vi "Field Get Field.vi"(6 "by sDisplayName? (f, by sFieldId)":bool, 7 "Include deleted? (F)":bool, 8 "error in (no error)":errorcluster, 9 "sFieldId or sDisplayName (\"\")":string, 10 "sxSequenceId (\"\")":string, 11 "Connection Refnum":T4) -> (0 "error out":errorcluster, 2 "Field":T1={"ixField"=0, "iSequenceOrder"=0, "sxFieldId"="", "sxSequenceId"="", "sDisplayName"="", "sValue"="", "sUnits"="", "nDataType"=enum."timestamp", "nNextItem"=enum."Reset", "fSystem"=FALSE, "fSystemValue"=FALSE, "fRequired"=FALSE, "fSetAtTest"=FALSE, "fTestField"=FALSE, "fDeleted"=FALSE, "fIndexed"=FALSE, "fFreeList"=FALSE}, 3 "Connection Refnum":T4, 4 "Data Present?":bool)   [LabVIEW 2011]
uses:
  Summitek EXT/ODBC/SQL Controls/Connection Refnum.ctl
  Field Record.ctl
  Field DataTypes.ctl
  Field NextItem.ctl
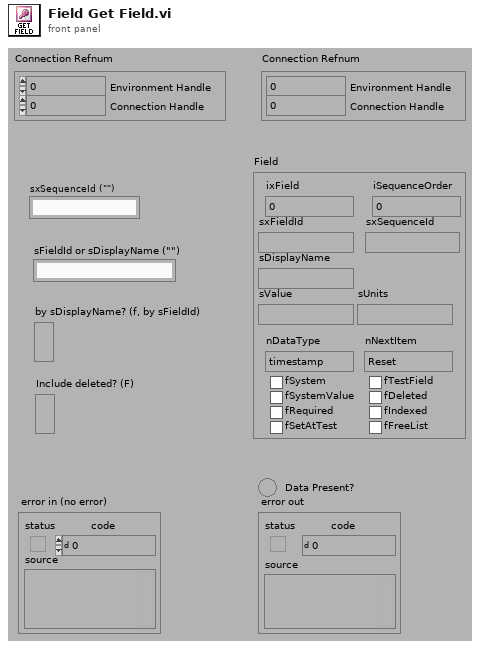
[diagram p1: front panel]
types:
  T1 = typedef "Field Record.ctl" = cluster{"ixField":i32, "iSequenceOrder":i32, "sxFieldId":string, "sxSequenceId":string, "sDisplayName":string, "sValue":string, "sUnits":string, "nDataType":T2, "nNextItem":T3, "fSystem":bool, "fSystemValue":bool, "fRequired":bool, "fSetAtTest":bool, "fTestField":bool, "fDeleted":bool, "fIndexed":bool, "fFreeList":bool}
  T2 = typedef "Field DataTypes.ctl" = enum32{"text", "numeric", "list", "timestamp", "boolean"}
  T3 = typedef "Field NextItem.ctl" = enum32{"Reset", "Retain", "Auto-Increment"}
  T4 = typedef "Connection Refnum.ctl" = cluster{"Environment Handle":i32, "Connection Handle":i32}
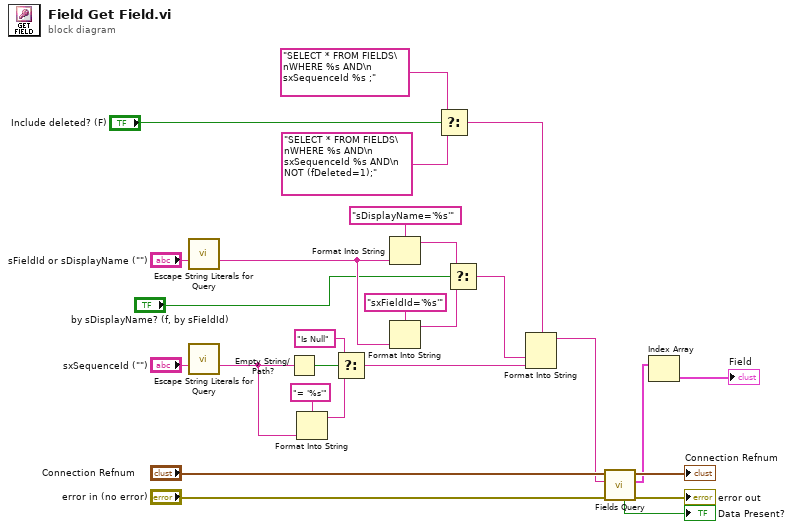
[diagram p0: block diagram]
diagram:
  n1 = call "Escape String Literals for Query.vi"("String"="sFieldId or sDisplayName (\"\")") -> ("escaped String"=w6:string)  [unwired: 1 in, 13 out]
  n2 = call "Escape String Literals for Query.vi"("String"="sxSequenceId (\"\")") -> ("escaped String"=w12:string)  [unwired: 1 in, 13 out]
  n3 = Empty String/Path?(string/path=w12) -> (empty?=w17:bool)
  n4 = Format Into String(format string="= '%s'", w12) -> (resulting string=w15:string)  [unwired: 2 in, 1 out]
  n5 = Select(t="Is Null", s=w17, f=w15) -> (s? t:f=w14:string)
  n6 = Format Into String(format string="sDisplayName='%s'", w6) -> (resulting string=w9:string)  [unwired: 2 in, 1 out]
  n7 = Format Into String(format string="sxFieldId='%s'", w6) -> (resulting string=w8:string)  [unwired: 2 in, 1 out]
  n8 = Select(t="SELECT * FROM FIELDS\nWHERE %s AND\n  sxSequenceId %s ;" ("Query Name"), s="Include deleted? (F)", f="SELECT * FROM FIELDS\nWHERE %s AND\n  sxSequenceId %s AND\n  NOT (fDeleted=1);" ("Query Name")) -> (s? t:f=w2:string)
  n9 = Select(t=w9, s="by sDisplayName? (f, by sFieldId)", f=w8) -> (s? t:f=w7:string)
  n10 = Format Into String(format string=w2, w7, w14) -> (resulting string=w25:string)  [unwired: 2 in, 1 out]
  n11 = call "Fields Query.vi"("error in (no error)"="error in (no error)", "Query"=w25, "Connection Refnum"="Connection Refnum") -> ("error out"=→"error out":errorcluster, "Fields"=w21:T1[], "Connection Refnum"=→"Connection Refnum":T4, "Data Present?"=→"Data Present?":bool)  [unwired: 2 in, 3 out]
  n12 = Index Array(array=w21) -> (element=→"Field":T1)  [unwired: 1 in]
